vi "UIM Tool.vi"(8 "Error In":errorcluster) -> (0 "Error Out":errorcluster)   [LabVIEW 2015]
doc: "Launch interactive window of the UI Manager Tool. This is the same tool that is launched from the tools menu in LabVIEW. \n\n<b>Note</b> - the execution of this VI is blocking, until the window is closed. It will suspend the execution of the code/thread you call it in."
uses:
  <vilib>/Utility/sysdir.llb/System Directory Type.ctl
  UIP/UIP.lvclass
  UIM.lvclass
panel:
  in  "Tab Control":enum32{"UI States", "UIP Definitions", "About"}(tab)
  in  "State Name":string="default"
  out "XML":string
  in  "Active Project Loaded VIs":u16(ring) items=["Capture UI State SubVI.vi", "UIM Tool.vi"]
  in  "Save":bool
  in  "Capture State":bool
  in  "Remove State":bool
  in  "Load":bool
  in  "Apply State":bool
  in  "States":u16(ring)
  in  "Refresh Button":bool
  in  "Save UIP List":bool=TRUE
  in  "Loaded UIPs":i32[](listbox)
  in  "Add UIP":bool
  in  "Remove UIP":bool
  in  "New UIP":bool
  in  "Reload UIPs":bool
  in  "Toggle Button":bool
  # "This tool is designed to help programmers capture and apply complex UI configurations to any LV VI, both edit and run-time.\nUsing the User Interface Manager Tool and its API you will be able to configure your UI any way you want, capture that configuration,\nexport and import it from XML file and apply any previously captured configuration at any moment. Thanks to this you can seperate\nthe configuration of your UIs from your application functionality and still be able to achieve any effect you could using standard\nVI Server methods and properties. \n\nIf the User Interface Property you want to capture is not handled by the standard provided UIPs, you can easily create a new one, using\nthe UIP Class Template. With this, by providing your own implementation for 5 simple menthods, you will be able to capture any property\nfrom any control in your VI.\n\nSome of the use cases that can be easily handled by this tool: localization of the UI, changing visibility of controls, changing the enabled\nstate of controls, changing the color scheme of the whole UI and many more...\n\nTo capture the state of UI quickly you can use the QuickDrop shortcut <Ctrl>+<U> or <Ctrl><Shift>+<U>. Status captured like this\nwill be saved to a file next to your VI, with the same name as your VI and the extension XML. You can load that file using this tool.\n\n\nhttps://www.ni.com/uim\n\n\n\n\n\n\n\n\n\n\n\n\n\nCreated by Piotr Kruczkowski"
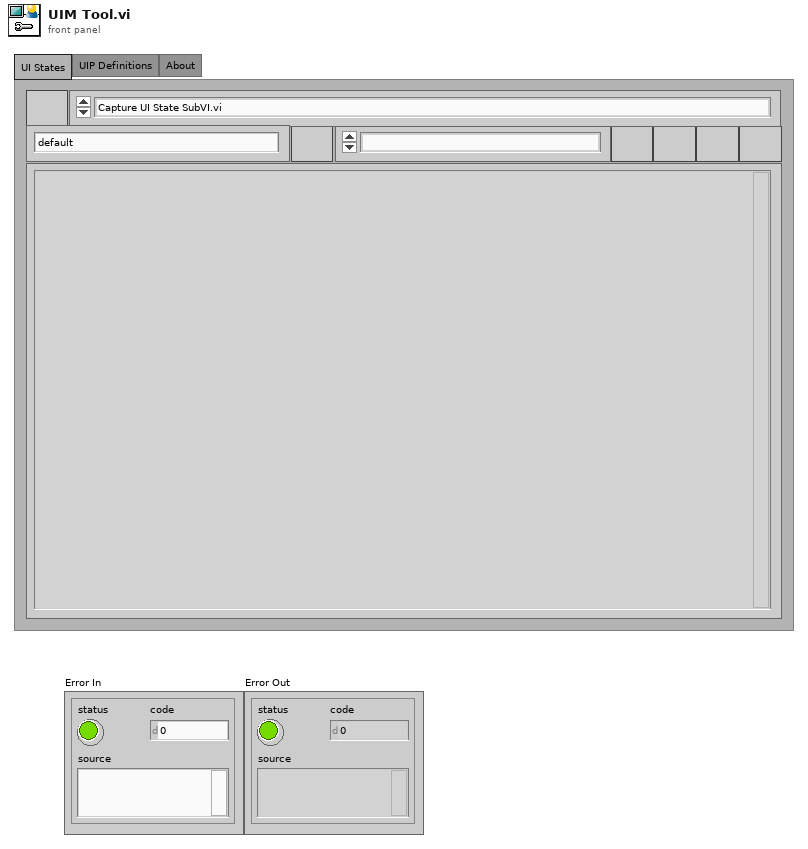
[diagram p1: front panel]
types:
  T1 = enum32{"Invalid", "Standard", "Closed", "Hidden", "Minimized", "Maximized"}
  T2 = typedef "System Directory Type.ctl" = i32
  T3 = typedef "LVPoint32TypeDef.ctl" = cluster{"Horizontal":i32, "Vertical":i32}
  T4 = typedef "LVRowAndColumnTypeDef.ctl" = cluster{"Row":i32, "Column":i32}
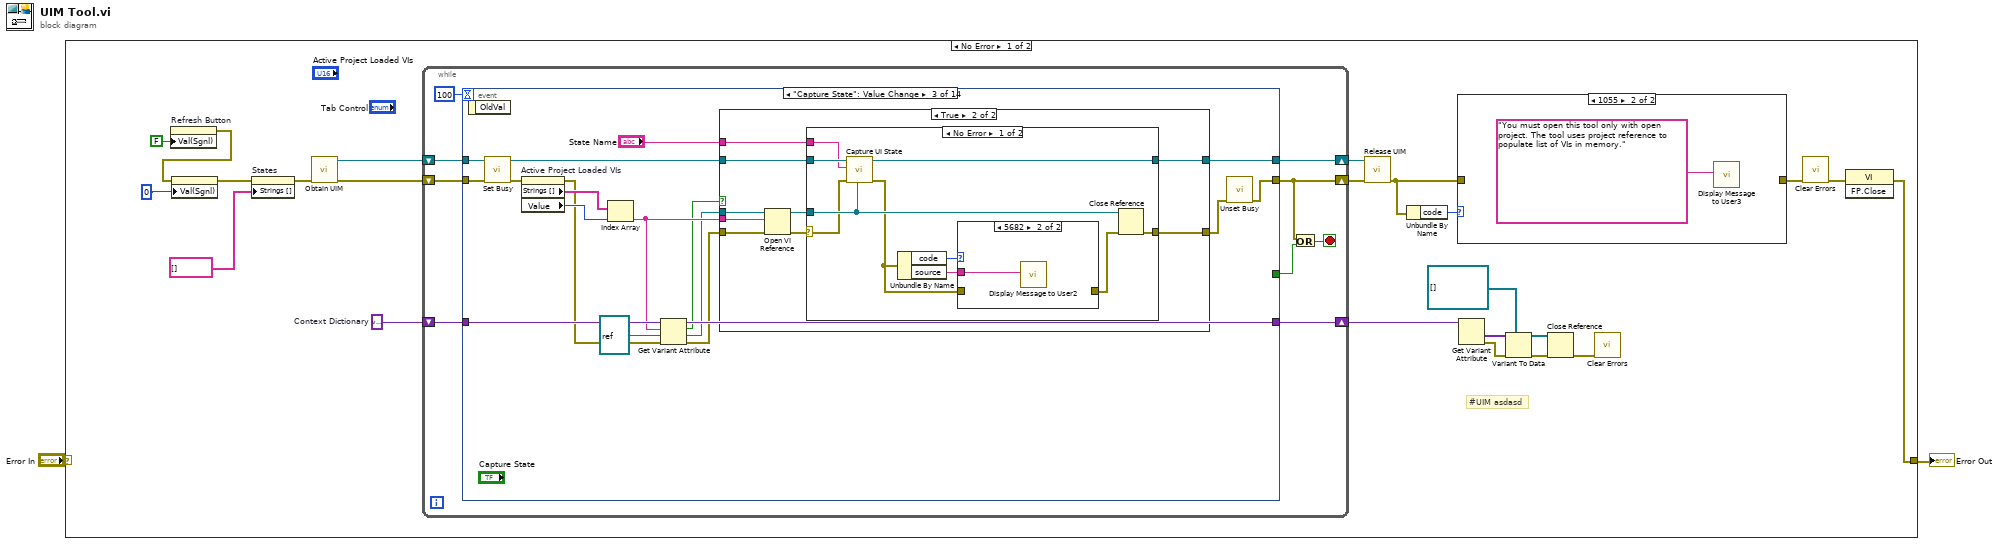
[diagram p0: block diagram]
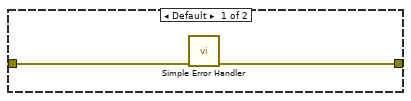
[diagram p2: hidden frame]
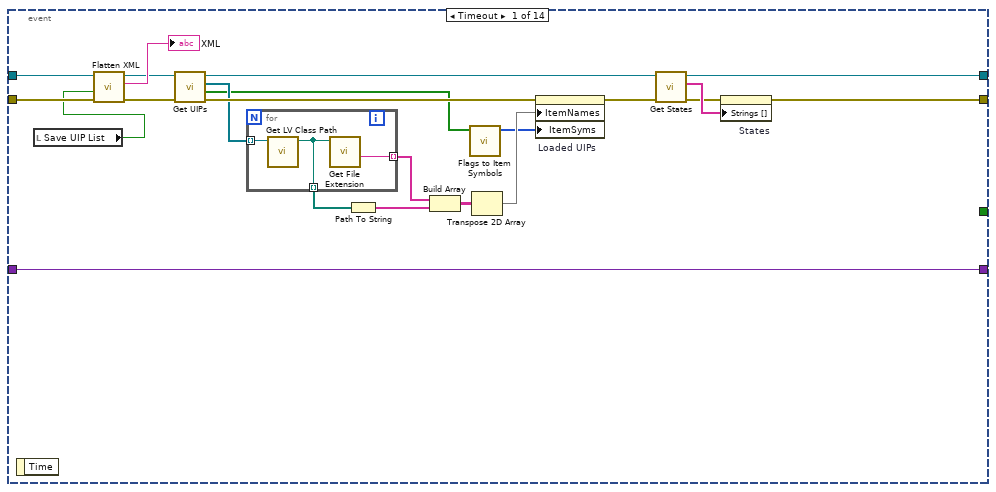
[diagram p3: hidden frame]
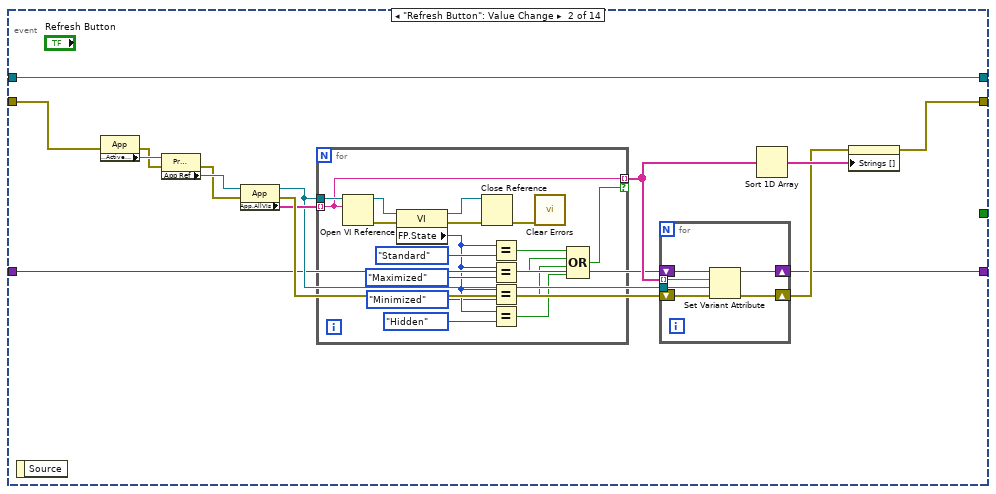
[diagram p4: hidden frame]
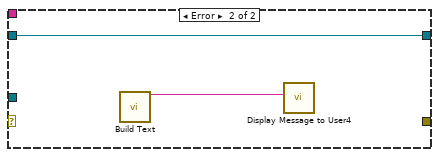
[diagram p7: hidden frame]
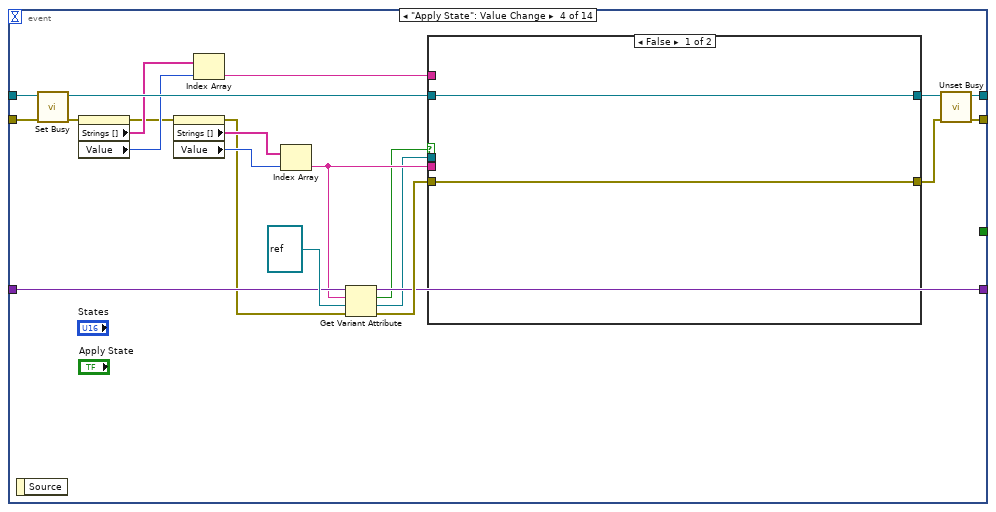
[diagram p8: hidden frame]
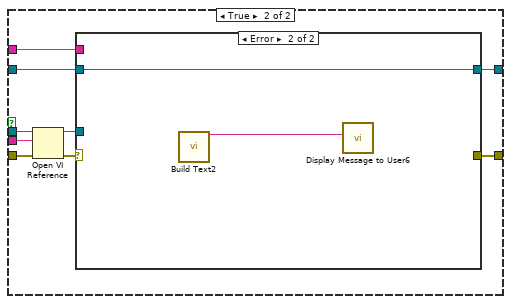
[diagram p9: hidden frame]
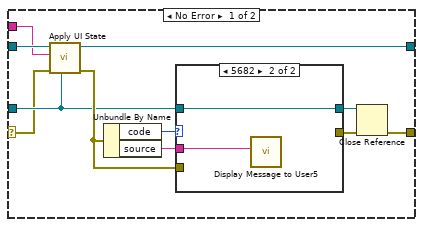
[diagram p10: hidden frame]
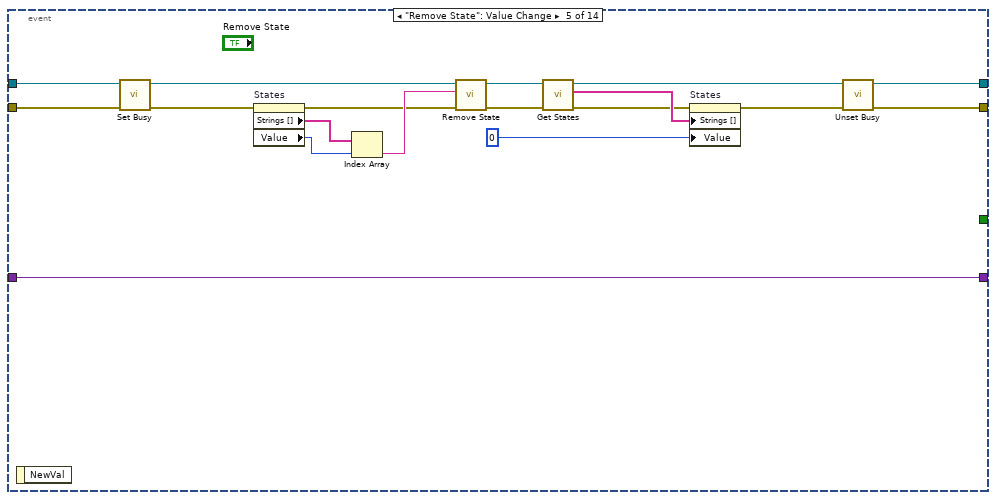
[diagram p12: hidden frame]
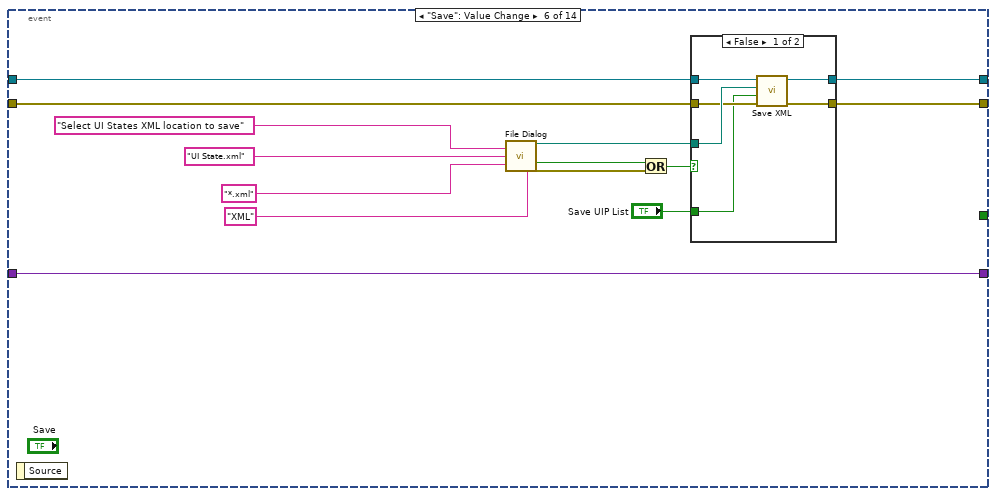
[diagram p13: hidden frame]
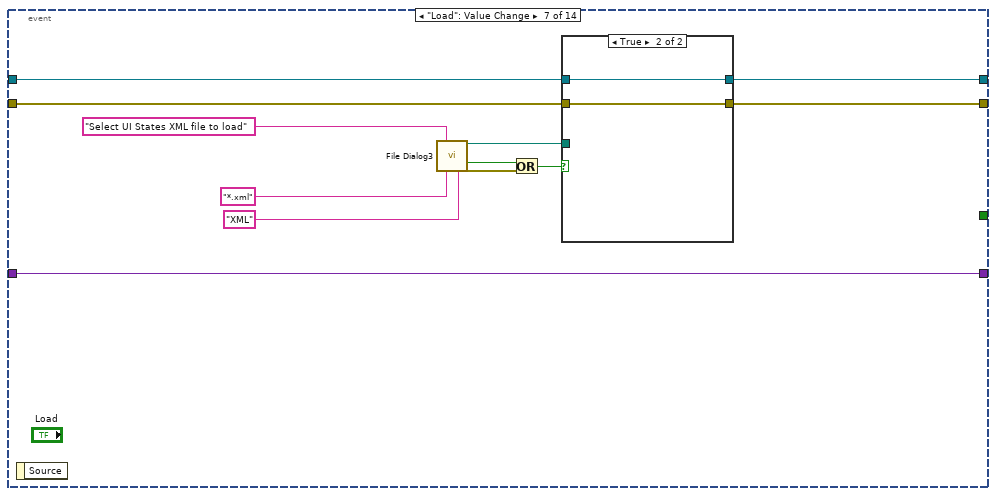
[diagram p15: hidden frame]
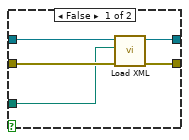
[diagram p16: hidden frame]
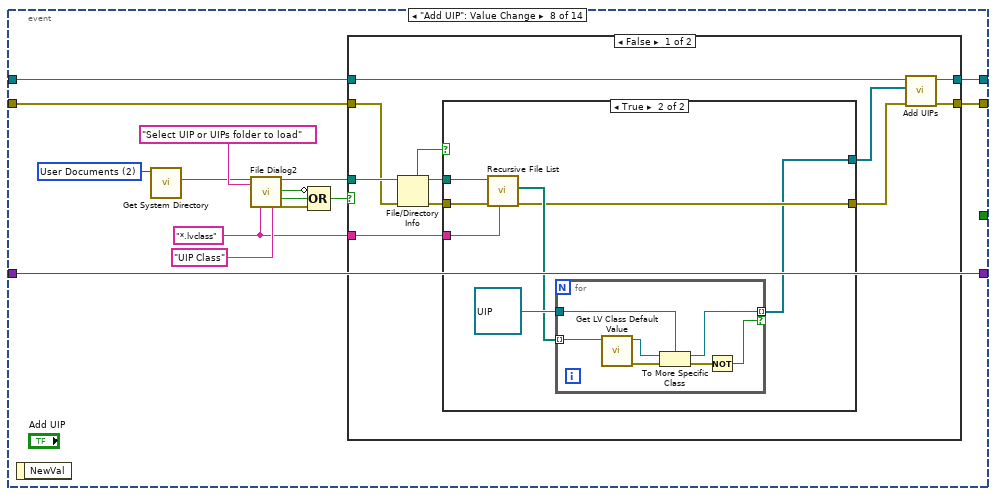
[diagram p17: hidden frame]
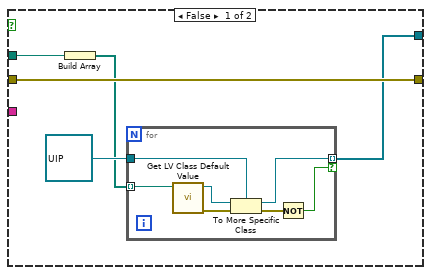
[diagram p18: hidden frame]
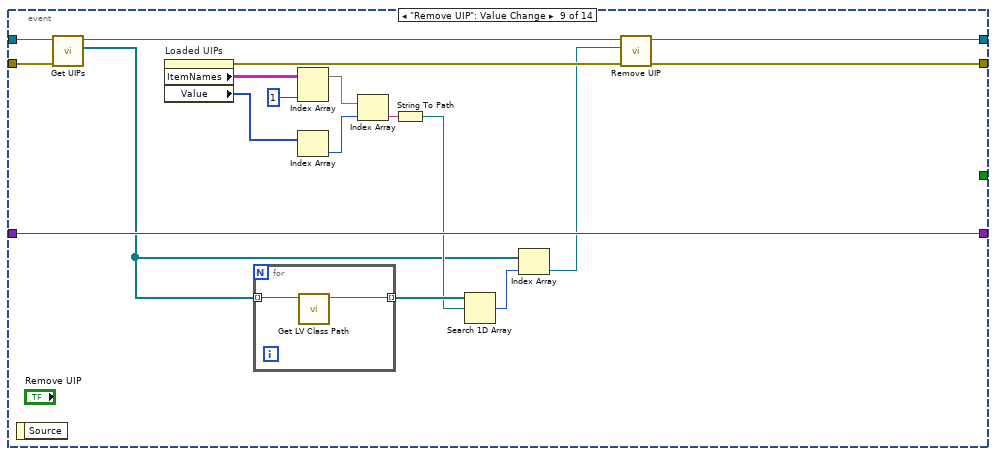
[diagram p20: hidden frame]
diagram:
  n1 = case shown="No Error" "Error In" {
    selector: "Error In" -> [_ w401]
    tunnel: [w7 w401] -> w1
    frame No Error {
      w19 = variant  # Context Dictionary
      # "#UIM asdasd"
      n2 = property on="Refresh Button" class="Bool (strict)"("Val(Sgnl)"=FALSE ("Value (Signaling)")) -> (error out=w4:errorcluster)  [unwired: 2 in, 1 out]
      n3 = property on="Active Project Loaded VIs" class="Ring (strict)"(error in=w4, "Val(Sgnl)"=u16 0 ("Value (Signaling)")) -> (error out=w22:errorcluster)  [unwired: 1 in, 1 out]
      n4 = property on="States" class="Ring (strict)"(error in=w22, "Strings []"=string[] []) -> (error out=w18:errorcluster)  [unwired: 1 in, 1 out]
      n5 = call "Obtain UIM.vi"("Error In"=w18) -> ("Error Out"=w5:errorcluster, "UIM Handle"=w6:refnum<data-value>)  [unwired: 9 in]
      n6 = while {
        shift-right: [w31] -> w23
        shift-left: w5 -> [w35]
        shift-right: [w34] -> w24
        shift-left: w6 -> [w37]
        shift-right: [w29] -> w17
        shift-left: w19 -> [w30]
        stop <- w32 stop-if-true
        n7 = event shown="[2] \"Capture State\": Value Change" {
          selector: _ -> [_ _ _ _ _ _ _ _ _ _ _ _ _ _]
          dyn-events: _ -> [_ _ _ _ _ _ _ _ _ _ _ _ _ _]
          timeout: 100 -> [_ _ _ _ _ _ _ _ _ _ _ _ _ _]
          tunnel: [_ _ _ _ _ _ _ _ _ _ _ w369 _ _] -> w33
          tunnel: w37 -> [w58 w77 w117 w162 w206 w220 w233 w257 w309 w327 w354 w367 w384 w399]
          tunnel: w35 -> [w56 w64 w112 w154 w199 w210 w230 w255 w308 w326 w353 w366 w383 w398]
          tunnel: [w49 w77 w115 w158 w196 w211 w232 w253 w317 w325 w357 w367 w371 w399] -> w34
          tunnel: [w38 w63 w109 w151 w192 w212 w231 w254 w316 w324 w358 w366 w372 w398] -> w31
          tunnel: w30 -> [w39 w66 w108 w149 w191 w208 w229 w250 w310 w322 w355 w365 w378 w392]
          tunnel: [w39 w65 w107 w145 w191 w208 w229 w250 w310 w322 w355 w365 w378 w392] -> w29
          event Timeout {
            n8 = event-data() -> ()  [unwired: 1 in, 1 out]
            n9 = local read "Save UIP List"() -> (w40:bool)
            n10 = call "Flatten XML.vi"("Error In"=w56, "Save UIP List (True)"=w40, "UIM In"=w58) -> ("Error Out"=w55:errorcluster, "XML"=→"XML":string, "UIM Out"=w57:refnum<data-value>)  [unwired: 6 in]
            n11 = call "Get UIPs.vi"("Error In"=w55, "UIM In"=w57) -> ("Error Out"=w54:errorcluster, "Enabled"=w42:bool[], "UIPs"=w45:refnum<class "UIP.lvclass">[], "UIM Out"=w52:refnum<data-value>)  [unwired: 6 in]
            n12 = for {
              tunnel: w45 -> [w61] mode=indexing
              tunnel: [w62] -> w44 mode=indexing
              tunnel: [w60] -> w41 mode=indexing
              n13 = call <vilib>:"Get LV Class Path.vi"("object"=w61) -> ("class path"=w60:path)  [unwired: 9 in, 1 out]
              n14 = call <vilib>:"Get File Extension.vi"("file"=w60) -> ("filename without extension"=w62:string)  [unwired: 6 in, 4 out]
            }
            n15 = Path To String(path=w41) -> (string=w48:string[])
            n16 = Build Array(w44, w48) -> (w47:string[][])
            n17 = call "Flags to Item Symbols.vi"("Flags"=w42) -> ("Item Symbols"=w43:i32[])  [unwired: 10 in]
            n18 = Transpose 2D Array(2D array=w47) -> (transposed array=w46:string[][])
            n19 = property on="Loaded UIPs" class="MCListbox (strict)"(error in=w54, "ItemNames"=w46, "ItemSyms"=w43) -> (error out=w51:errorcluster)  [unwired: 1 in, 1 out]
            n20 = call "Get States.vi"("Error In"=w51, "UIM In"=w52) -> ("Error Out"=w50:errorcluster, "States"=w53:string[], "UIM Out"=w49:refnum<data-value>)  [unwired: 7 in]
            n21 = property on="States" class="Ring (strict)"(error in=w50, "Strings []"=w53) -> (error out=w38:errorcluster)  [unwired: 1 in, 1 out]
          }
          event "Refresh Button": Value Change {
            n22 = event-data() -> ()  [unwired: 1 in, 1 out]
            n23 = property class="App"(error in=w64) -> (error out=w74:errorcluster, "Project.ActiveProject"=w76:refnum<vi>)  [unwired: 1 in, 1 out]
            n24 = property class="Project"(reference=w76, error in=w74) -> (error out=w73:errorcluster, "App Ref"=w75:refnum<vi>)  [unwired: 1 out]
            n25 = property class="App"(reference=w75, error in=w73) -> (reference out=w68:refnum<vi>, error out=w71:errorcluster, "App.AllVIs"=w69:string[])
            n26 = for {
              tunnel: w69 -> [w80] mode=indexing
              tunnel: w68 -> [w81]
              tunnel: [w80] -> w67 mode=indexing if=w79
              n27 = Open VI Reference(application reference (local)=w81, vi path=w80) -> (vi reference=w93:refnum<vi>, error out=w94:errorcluster)  [unwired: 4 in]
              n28 = property class="VI"(reference=w93, error in=w94) -> (reference out=w82:refnum<vi>, error out=w83:errorcluster, "FP.State"=w88:T1)
              n29 = Close Reference(reference=w82, error in (no error)=w83) -> (error out=w78:errorcluster)
              n30 = Equal?(x=w88, y=T1."Standard") -> (x = y?=w91:bool)
              n31 = Equal?(x=w88, y=T1."Maximized") -> (x = y?=w86:bool)
              n32 = Equal?(x=w88, y=T1."Minimized") -> (x = y?=w85:bool)
              n33 = Equal?(x=w88, y=T1."Hidden") -> (x = y?=w84:bool)
              n34 = call <vilib>:"Clear Errors.vi"("error in (no error)"=w78) -> ()  [unwired: 5 in, 2 out]
              n35 = Compound Arithmetic op=OR(w91, w86, w85, w84) -> (w79:bool)
            }
            n36 = for {
              tunnel: w68 -> [w99]
              tunnel: w67 -> [w98] mode=indexing
              shift-right: [w97] -> w70
              shift-left: w71 -> [w96]
              shift-right: [w95] -> w65
              shift-left: w66 -> [w100]
              n37 = Set Variant Attribute(Variant=w100, name=w98, value=w99, error in=w96) -> (Variant out=w95:variant, error out=w97:errorcluster)  [unwired: 1 out]
            }
            n38 = Sort 1D Array(array=w67) -> (sorted array=w72:string[])
            n39 = property on="Active Project Loaded VIs" class="Ring (strict)"(error in=w70, "Strings []"=w72) -> (error out=w63:errorcluster)  [unwired: 1 in, 1 out]
          }
          event "Capture State": Value Change {
            n40 = event-data() -> ()  [unwired: 1 in, 1 out]
            n41 = call <vilib>:"Set Busy.vi"("error in (no error)"=w112) -> ("error out"=w111:errorcluster)  [unwired: 9 in, 1 out]
            n42 = property on="Active Project Loaded VIs" class="Ring (strict)"(error in=w111) -> (error out=w104:errorcluster, "Strings []"=w114:string[], "Value"=w113:u16)  [unwired: 1 in, 1 out]
            n43 = Index Array(array=w114, index=w113) -> (element=w106:string)
            n44 = Get Variant Attribute(Variant=w108, name=w106, default value (empty Variant)=refnum<vi> refnum ("reference out"), error in=w104) -> (duplicate Variant=w107:variant, found=w102:bool, value=w101:refnum<vi>, error out=w103:errorcluster)
            n45 = case shown="True" w102 {
              tunnel: w117 -> [w119 w128]
              tunnel: "State Name" -> [_ w127]
              tunnel: [w119 w126] -> w115
              tunnel: [w118 w125] -> w110
              tunnel: w106 -> [_ w123]
              tunnel: w103 -> [w118 w121]
              tunnel: w101 -> [_ w122]
              frame False {
                # "Application reference not found for this VI\nname. Dont do anything."
              }
              frame True {
                n46 = Open VI Reference(application reference (local)=w122, vi path=w123, error in (no error)=w121) -> (vi reference=w124:refnum<vi>, error out=w120:errorcluster)  [unwired: 3 in]
                n47 = case shown="No Error" w120 {
                  selector: w120 -> [w129 _]
                  tunnel: w128 -> [w138 w142]
                  tunnel: w127 -> [w137 _]
                  tunnel: [w136 w142] -> w126
                  tunnel: [w135 _] -> w125
                  tunnel: w124 -> [w134 _]
                  frame No Error {
                    n48 = call "Capture UI State.vi"("VI Ref (Calling VI)"=w134, "Error In"=w129, "State Name"=w137, "UIM In"=w138) -> ("Error Out"=w131:errorcluster, "UIM Out"=w136:refnum<data-value>)  [unwired: 6 in]
                    n49 = Unbundle By Name(w131) -> ("code"=w133:i32, "source"=w130:string)
                    n50 = case shown="5682" w133 {
                      tunnel: [w139 _] -> w132
                      tunnel: w131 -> [w139 _]
                      tunnel: w130 -> [_ w140]
                      frame Default {
                      }
                      frame 5682 {
                        n51 = call "Display Message to User2"("Message"=w140) -> ()  [unwired: 9 in, 2 out]
                      }
                    }
                    n52 = Close Reference(reference=w134, error in (no error)=w132) -> (error out=w135:errorcluster)
                  }
                  frame Error {
                    n53 = call "Build Text"() -> ("Result"=w141:string)  [unwired: 14 in, 1 out]
                    n54 = call "Display Message to User4"("Message"=w141) -> ()  [unwired: 9 in, 2 out]
                  }
                }
              }
            }
            n55 = call <vilib>:"Unset Busy.vi"("error in (no error)"=w110) -> ("error out"=w109:errorcluster)  [unwired: 10 in]
          }
          event "Apply State": Value Change {
            n56 = event-data() -> ()  [unwired: 1 in, 1 out]
            n57 = call <vilib>:"Set Busy.vi"("error in (no error)"=w154) -> ("error out"=w153:errorcluster)  [unwired: 9 in, 1 out]
            n58 = property on="States" class="Ring (strict)"(error in=w153) -> (error out=w159:errorcluster, "Strings []"=w161:string[], "Value"=w160:u16)  [unwired: 1 in, 1 out]
            n59 = property on="Active Project Loaded VIs" class="Ring (strict)"(error in=w159) -> (error out=w148:errorcluster, "Strings []"=w156:string[], "Value"=w157:u16)  [unwired: 1 in, 1 out]
            n60 = Index Array(array=w161, index=w160) -> (element=w155:string)
            n61 = Index Array(array=w156, index=w157) -> (element=w147:string)
            n62 = Get Variant Attribute(Variant=w149, name=w147, default value (empty Variant)=refnum<vi> refnum ("reference out"), error in=w148) -> (duplicate Variant=w145:variant, found=w143:bool, value=w144:refnum<vi>, error out=w146:errorcluster)
            n63 = case shown="False" w143 {
              tunnel: w162 -> [w164 w173]
              tunnel: [w164 w172] -> w158
              tunnel: [w163 w171] -> w152
              tunnel: w147 -> [_ w170]
              tunnel: w144 -> [_ w167]
              tunnel: w146 -> [w163 w168]
              tunnel: w155 -> [_ w169]
              frame False {
              }
              frame True {
                n64 = Open VI Reference(application reference (local)=w167, vi path=w170, error in (no error)=w168) -> (vi reference=w166:refnum<vi>, error out=w165:errorcluster)  [unwired: 3 in]
                n65 = case shown="Error" w165 {
                  selector: w165 -> [w174 _]
                  tunnel: w173 -> [w184 w190]
                  tunnel: [w183 w190] -> w172
                  tunnel: [w182 _] -> w171
                  tunnel: w169 -> [w181 _]
                  tunnel: w166 -> [w176 _]
                  frame No Error {
                    n66 = call "Apply UI State.vi"("VI Ref (Calling VI)"=w176, "Error In"=w174, "State Name"=w181, "UIM In"=w184) -> ("Error Out"=w178:errorcluster, "UIM Out"=w183:refnum<data-value>)  [unwired: 6 in]
                    n67 = Unbundle By Name(w178) -> ("code"=w179:i32, "source"=w180:string)
                    n68 = case shown="5682" w179 {
                      tunnel: [w186 _] -> w177
                      tunnel: w178 -> [w186 _]
                      tunnel: w180 -> [_ w188]
                      tunnel: w176 -> [w185 w187]
                      tunnel: [w185 w187] -> w175
                      frame Default {
                      }
                      frame 5682 {
                        n69 = call "Display Message to User5"("Message"=w188) -> ()  [unwired: 9 in, 2 out]
                      }
                    }
                    n70 = Close Reference(reference=w175, error in (no error)=w177) -> (error out=w182:errorcluster)
                  }
                  frame Error {
                    n71 = call "Build Text2"() -> ("Result"=w189:string)  [unwired: 14 in, 1 out]
                    n72 = call "Display Message to User6"("Message"=w189) -> ()  [unwired: 9 in, 2 out]
                  }
                }
              }
            }
            n73 = call <vilib>:"Unset Busy.vi"("error in (no error)"=w152) -> ("error out"=w151:errorcluster)  [unwired: 10 in]
          }
          event "Remove State": Value Change {
            n74 = event-data() -> ()  [unwired: 1 in, 1 out]
            n75 = call <vilib>:"Set Busy.vi"("error in (no error)"=w199) -> ("error out"=w193:errorcluster)  [unwired: 9 in, 1 out]
            n76 = property on="States" class="Ring (strict)"(error in=w193) -> (error out=w198:errorcluster, "Strings []"=w203:string[], "Value"=w202:u16)  [unwired: 1 in, 1 out]
            n77 = Index Array(array=w203, index=w202) -> (element=w201:string)
            n78 = call "Remove State.vi"("Error In"=w198, "State"=w201, "UIM In"=w206) -> ("Error Out"=w197:errorcluster, "UIM Out"=w205:refnum<data-value>)  [unwired: 7 in]
            n79 = call "Get States.vi"("Error In"=w197, "UIM In"=w205) -> ("Error Out"=w195:errorcluster, "States"=w204:string[], "UIM Out"=w196:refnum<data-value>)  [unwired: 7 in]
            n80 = property on="States" class="Ring (strict)"(error in=w195, "Strings []"=w204, "Value"=0) -> (error out=w194:errorcluster)  [unwired: 1 in, 1 out]
            n81 = call <vilib>:"Unset Busy.vi"("error in (no error)"=w194) -> ("error out"=w192:errorcluster)  [unwired: 10 in]
          }
          event "Save": Value Change {
            n82 = event-data() -> ()  [unwired: 1 in, 1 out]
            n83 = call "File Dialog"("prompt"="Select UI States XML location to save", "default name"="UI State.xml", "pattern (all files)"="*.xml", "pattern label"="XML") -> ("selected path"=w216:path, "cancelled"=w218:bool, "error out"=w219:errorcluster)  [unwired: 8 in, 1 out]
            n84 = Or(x=w218, y=w219) -> (x .or. y?=w217:bool)
            n85 = case shown="False" w217 {
              tunnel: w220 -> [w226 w228]
              tunnel: w216 -> [w225 _]
              tunnel: w210 -> [w224 w227]
              tunnel: [w223 w227] -> w212
              tunnel: [w222 w228] -> w211
              tunnel: "Save UIP List" -> [w221 _]
              frame False {
                n86 = call "Save XML.vi"("Error In"=w224, "Save UIP List (True)"=w221, "UIM XML Path"=w225, "UIM In"=w226) -> ("Error Out"=w223:errorcluster, "UIM Out"=w222:refnum<data-value>)  [unwired: 6 in]
              }
              frame True {
              }
            }
          }
          event "Load": Value Change {
            n87 = event-data() -> ()  [unwired: 1 in, 1 out]
            n88 = call "File Dialog3"("prompt"="Select UI States XML file to load", "pattern (all files)"="*.xml", "pattern label"="XML") -> ("selected path"=w237:path, "cancelled"=w239:bool, "error out"=w240:errorcluster)  [unwired: 9 in, 1 out]
            n89 = Or(x=w239, y=w240) -> (x .or. y?=w238:bool)
            n90 = case shown="True" w238 {
              tunnel: w233 -> [w241 w247]
              tunnel: w237 -> [w242 _]
              tunnel: w230 -> [w244 w246]
              tunnel: [w243 w246] -> w231
              tunnel: [w245 w247] -> w232
              frame False {
                n91 = call "Load XML.vi"("Error In"=w244, "XML File"=w242, "UIM In"=w241) -> ("Error Out"=w243:errorcluster, "UIM Out"=w245:refnum<data-value>)  [unwired: 7 in]
              }
              frame True {
              }
            }
          }
          event "Add UIP": Value Change {
            w249 = T2 2 items=["User Home"=0, "User Desktop"=1, "User Documents"=2, "User Application Data"=3, "User Preferences"=4, "User Temporary"=5, "Public Documents"=6, "Public Application Data"=7, "Public Preferences"=8, "Public Cache"=13, "System Core Libraries"=9, "System Installed Libraries"=10, "Application Files"=11, "Boot Volume Root"=12] ("system directory type")
            w251 = "*.lvclass" ("pattern (all files)")
            n92 = event-data() -> ()  [unwired: 1 in, 1 out]
            n93 = call <vilib>:"Get System Directory.vi"("system directory type"=w249) -> ("system directory"=w248:path)  [unwired: 10 in]
            n94 = call "File Dialog2"("start path"=w248, "prompt"="Select UIP or UIPs folder to load", "pattern (all files)"=w251, "pattern label"="UIP Class") -> ("selected path"=w256:path, "exists"=w252:bool, "cancelled"=w259:bool, "error out"=w260:errorcluster)  [unwired: 8 in]
            n95 = Compound Arithmetic op=OR(invert w252, w259, w260) -> (w258:bool)
            n96 = case shown="False" w258 {
              tunnel: w257 -> [w273 w301]
              tunnel: w256 -> [w268 _]
              tunnel: w255 -> [w265 w300]
              tunnel: [w272 w300] -> w254
              tunnel: [w271 w301] -> w253
              tunnel: w251 -> [w270 _]
              frame False {
                n97 = File/Directory Info(path=w268, error in=w265) -> (path out=w266:path, directory=w267:bool, error out=w264:errorcluster)  [unwired: 4 out]
                n98 = case shown="True" w267 {
                  tunnel: w270 -> [_ w292]
                  tunnel: [w274 w287] -> w269
                  tunnel: w266 -> [w278 w291]
                  tunnel: w264 -> [w277 w286]
                  tunnel: [w277 w288] -> w263
                  frame False {
                    n99 = Build Array(w278) -> (w275:path[])
                    n100 = for {
                      tunnel: w275 -> [w285] mode=indexing
                      tunnel: [w282] -> w274 mode=indexing if=w280
                      tunnel: refnum<class "UIP.lvclass"> refnum ("UIP") -> [w279]
                      n101 = call <vilib>:"Get LV Class Default Value.vi"("class path"=w285) -> ("error out"=w284:errorcluster, "object"=w283:refnum<class>)  [unwired: 9 in]
                      n102 = To More Specific Class(target class=w279, reference=w283, error in=w284) -> (specific class reference=w282:refnum<class "UIP.lvclass">, error out=w281:errorcluster)
                      n103 = Not(x=w281) -> (.not. x?=w280:bool)
                    }
                  }
                  frame True {
                    n104 = call <vilib>:"Recursive File List.vi"("pattern"=w292, "error in (no error)"=w286, "Folder Path"=w291) -> ("error out"=w288:errorcluster, "All Files in Dir"=w289:path[])  [unwired: 4 in, 3 out]
                    n105 = for {
                      tunnel: w289 -> [w299] mode=indexing
                      tunnel: [w296] -> w287 mode=indexing if=w294
                      tunnel: refnum<class "UIP.lvclass"> refnum ("UIP") -> [w293]
                      n106 = call <vilib>:"Get LV Class Default Value.vi"("class path"=w299) -> ("error out"=w298:errorcluster, "object"=w297:refnum<class>)  [unwired: 9 in]
                      n107 = To More Specific Class(target class=w293, reference=w297, error in=w298) -> (specific class reference=w296:refnum<class "UIP.lvclass">, error out=w295:errorcluster)
                      n108 = Not(x=w295) -> (.not. x?=w294:bool)
                    }
                  }
                }
                n109 = call "Add UIPs.vi"("Error In"=w263, "UIPs"=w269, "UIM In"=w273) -> ("Error Out"=w272:errorcluster, "UIM Out"=w271:refnum<data-value>)  [unwired: 7 in]
              }
              frame True {
              }
            }
          }
          event "Remove UIP": Value Change {
            n110 = event-data() -> ()  [unwired: 1 in, 1 out]
            n111 = call "Get UIPs.vi"("Error In"=w308, "UIM In"=w309) -> ("UIPs"=w304:refnum<class "UIP.lvclass">[], "UIM Out"=w307:refnum<data-value>)  [unwired: 6 in, 2 out]
            n112 = property on="Loaded UIPs" class="MCListbox (strict)"() -> (error out=w315:errorcluster, "ItemNames"=w319:string[][], "Value"=w312:i32[])  [unwired: 2 in, 1 out]
            n113 = for {
              tunnel: w304 -> [w321] mode=indexing
              tunnel: [w320] -> w306 mode=indexing
              n114 = call <vilib>:"Get LV Class Path.vi"("object"=w321) -> ("class path"=w320:path)  [unwired: 9 in, 1 out]
            }
            n115 = Index Array(array=w319, index (col)=1 ("disabled index (col)")) -> (element=w314:string[])  [unwired: 1 in]
            n116 = Index Array(array=w312) -> (element=w311:i32)  [unwired: 1 in]
            n117 = Index Array(array=w314, index=w311) -> (element=w318:string)
            n118 = String To Path(string=w318) -> (path=w305:path)
            n119 = Search 1D Array(1D array=w306, element=w305) -> (index of element=w303:i32)  [unwired: 1 in]
            n120 = Index Array(array=w304, index=w303) -> (element=w302:refnum<class "UIP.lvclass">)
            n121 = call "Remove UIP.vi"("Error In"=w315, "UIP"=w302, "UIM In"=w307) -> ("Error Out"=w316:errorcluster, "UIM Out"=w317:refnum<data-value>)  [unwired: 7 in]
          }
          event "Loaded UIPs": Mouse Down {
            n122 = event-data() -> ("Coords"=w330:T3)  [unwired: 1 in]
            n123 = invoke on="Loaded UIPs" class="MCListbox (strict)" method="Point To Row Column"("Point"=w330) -> ("InBounds"=w323:bool, "CellPosition"=w329:T4)  [unwired: 6 in, 5 out]
            n124 = Unbundle By Name(w329) -> ("Row"=w328:i32)
            n125 = case shown="True" w323 {
              tunnel: w328 -> [_ w343]
              tunnel: w327 -> [w332 w340]
              tunnel: w326 -> [w331 w339]
              tunnel: [w332 w337] -> w325
              tunnel: [w331 w336] -> w324
              frame False {
              }
              frame True {
                n126 = property on="Loaded UIPs" class="MCListbox (strict)"() -> ("ItemSyms"=w341:i32[])  [unwired: 2 in, 2 out]
                n127 = in-place {
                  w347 = 38
                  n128 = in-place-array #1(w341, w343) -> (w345:i32)
                  n129 = Equal?(x=w345, y=w347) -> (x = y?=w348:bool)
                  n130 = Select(t=37, s=w348, f=w347) -> (s? t:f=w344:i32)
                  n131 = in-place-array #1(w344) -> (w342:i32[])  [unwired: 1 out]
                }
                n132 = call "Get UIPs.vi"("Error In"=w339, "UIM In"=w340) -> ("Error Out"=w335:errorcluster, "UIPs"=w333:refnum<class "UIP.lvclass">[], "UIM Out"=w338:refnum<data-value>)  [unwired: 6 in, 1 out]
                n133 = call "Items Symbols to Flags.vi"("Item Symbols"=w342) -> ("Flags"=w334:bool[])  [unwired: 10 in]
                n134 = property on="Loaded UIPs" class="MCListbox (strict)"("ItemSyms"=w342) -> ()  [unwired: 2 in, 2 out]
                n135 = call "Add UIPs.vi"("Error In"=w335, "Enabled (True)"=w334, "UIPs"=w333, "UIM In"=w338) -> ("Error Out"=w336:errorcluster, "UIM Out"=w337:refnum<data-value>)  [unwired: 6 in]
              }
            }
          }
          event "Toggle Button": Value Change {
            n136 = event-data() -> ()  [unwired: 1 in, 1 out]
            n137 = property on="Loaded UIPs" class="MCListbox (strict)"() -> ("ItemSyms"=w359:i32[])  [unwired: 2 in, 2 out]
            n138 = for {
              tunnel: w359 -> [w361] mode=indexing
              tunnel: [w360] -> w356 mode=indexing
              w363 = 38
              n139 = Equal?(x=w361, y=w363) -> (x = y?=w364:bool)
              n140 = Select(t=37, s=w364, f=w363) -> (s? t:f=w360:i32)
            }
            n141 = call "Get UIPs.vi"("Error In"=w353, "UIM In"=w354) -> ("Error Out"=w349:errorcluster, "UIPs"=w350:refnum<class "UIP.lvclass">[], "UIM Out"=w352:refnum<data-value>)  [unwired: 6 in, 1 out]
            n142 = call "Items Symbols to Flags.vi"("Item Symbols"=w356) -> ("Flags"=w351:bool[])  [unwired: 10 in]
            n143 = property on="Loaded UIPs" class="MCListbox (strict)"("ItemSyms"=w356) -> ()  [unwired: 2 in, 2 out]
            n144 = call "Add UIPs.vi"("Error In"=w349, "Enabled (True)"=w351, "UIPs"=w350, "UIM In"=w352) -> ("Error Out"=w358:errorcluster, "UIM Out"=w357:refnum<data-value>)  [unwired: 6 in]
          }
          event Panel Close? {
            n145 = event-data() -> ()  [unwired: 1 in, 1 out]
            n146 = call "Display Message to User"("Message"="Are you sure you want to quit?") -> ("Yes"=w369:bool)  [unwired: 9 in, 1 out]
            n147 = Not(x=w369) -> (.not. x?=w370:bool)
            n148 = event-data("Discard?"=w370) -> ()  [unwired: 1 in, 1 out]
          }
          event "Reload UIPs": Value Change {
            n149 = event-data() -> ()  [unwired: 1 in, 1 out]
            n150 = call "Get UIPs.vi"("Error In"=w383, "UIM In"=w384) -> ("Error Out"=w381:errorcluster, "UIPs"=w380:refnum<class "UIP.lvclass">[], "UIM Out"=w382:refnum<data-value>)  [unwired: 6 in, 1 out]
            n151 = for {
              shift-right: [w387] -> w377
              shift-left: w381 -> [w388]
              tunnel: w380 -> [w386] mode=indexing
              shift-right: [w385] -> w379
              shift-left: w382 -> [w389]
              n152 = call "Remove UIP.vi"("Error In"=w388, "UIP"=w386, "UIM In"=w389) -> ("Error Out"=w387:errorcluster, "UIM Out"=w385:refnum<data-value>)  [unwired: 7 in]
            }
            n153 = call "Get Default UIPs.vi"() -> ("UIPs"=w376:refnum<class "UIP.lvclass">[])  [unwired: 11 in]
            n154 = call "Add UIPs.vi"("Error In"=w377, "UIPs"=w376, "UIM In"=w379) -> ("Error Out"=w374:errorcluster, "UIM Out"=w375:refnum<data-value>)  [unwired: 7 in]
            n155 = call "Get Plugin UIPs.vi"() -> ("UIPs"=w373:refnum<class "UIP.lvclass">[])  [unwired: 11 in]
            n156 = call "Add UIPs.vi"("Error In"=w374, "UIPs"=w373, "UIM In"=w375) -> ("Error Out"=w372:errorcluster, "UIM Out"=w371:refnum<data-value>)  [unwired: 7 in]
          }
          event "New UIP": Value Change {
            w391 = T2 2 items=["User Home"=0, "User Desktop"=1, "User Documents"=2, "User Application Data"=3, "User Preferences"=4, "User Temporary"=5, "Public Documents"=6, "Public Application Data"=7, "Public Preferences"=8, "Public Cache"=13, "System Core Libraries"=9, "System Installed Libraries"=10, "Application Files"=11, "Boot Volume Root"=12] ("system directory type")
            n157 = event-data() -> ()  [unwired: 1 in, 1 out]
            n158 = call <vilib>:"Get System Directory.vi"("system directory type"=w391) -> ("system directory"=w390:path)  [unwired: 10 in]
            n159 = call "File Dialog4"("start path"=w390, "prompt"="Select location for Template UIP copy") -> ("selected path"=w393:path, "cancelled"=w395:bool, "error out"=w396:errorcluster)  [unwired: 10 in, 1 out]
            n160 = Or(x=w395, y=w396) -> (x .or. y?=w394:bool)
            n161 = case shown="False" w394 {
              tunnel: w393 -> [w400 _]
              frame False {
                n162 = call "Copy Template UIP.vi"("Dest Path"=w400) -> ()  [unwired: 9 in, 2 out]
              }
              frame True {
              }
            }
          }
        }
        n163 = Or(x=w31, y=w33) -> (x .or. y?=w32:bool)
      }
      n164 = call "Release UIM.vi"("Error In"=w23, "UIM Handle"=w24) -> ("Error Out"=w9:errorcluster)  [unwired: 9 in]
      n165 = Unbundle By Name(w9) -> ("code"=w10:i32)
      n166 = case shown="1055" w10 {
        tunnel: w9 -> [w27 _]
        tunnel: [w26 _] -> w8
        frame Default {
          n167 = call <vilib>:"Simple Error Handler.vi"("error in (no error)"=w27) -> ("error out"=w26:errorcluster)  [unwired: 4 in, 4 out]
        }
        frame 1055 {
          n168 = call "Display Message to User3"("Message"="You must open this tool only with open project. The tool uses project reference to populate list of VIs in memory.") -> ()  [unwired: 9 in, 2 out]
        }
      }
      n169 = Get Variant Attribute(Variant=w17) -> (values=w16:variant[], error out=w12:errorcluster)  [unwired: 3 in, 2 out]
      n170 = Variant To Data(error in=w12, type=refnum<vi>[] [] ("reference out"), Variant=w16) -> (data=w14:refnum<vi>[], error out=w13:errorcluster)
      n171 = Close Reference(reference=w14, error in (no error)=w13) -> (error out=w11:errorcluster)
      n172 = call <vilib>:"Clear Errors.vi"("error in (no error)"=w11) -> ()  [unwired: 5 in, 2 out]
      n173 = call <vilib>:"Clear Errors.vi"("error in (no error)"=w8) -> ("error out"=w20:errorcluster)  [unwired: 5 in, 1 out]
      n174 = invoke class="VI" method="FP.Close"(error in=w20) -> (error out=w7:errorcluster)  [unwired: 2 in, 2 out]
    }
    frame Error {
    }
  }
  "Error Out" <- w1
